vi "Vision Processing.vi"(4 "error in (no error)":errorcluster, 7 "Image Size":T3=enum."320x240") -> ()   [LabVIEW 2015]
uses:
  Vision Support Code/Camera Types.ctl
  <vilib>/Rock Robotics/WPI/Camera/WPI_CameraImageSize.ctl
  <vilib>/Rock Robotics/WPI/Camera/WPI_CameraWhite Balance Values.ctl
  <vilib>/Rock Robotics/WPI/Camera/WPI_CameraExposure Values.ctl
  <vilib>/Rock Robotics/WPI/Camera/WPI_CameraFrameRate.ctl
  Robot Global Data.vi
  <vilib>/vision/NI_Vision_Development_Module.lvlib
panel:
  out "Highest Avg Score":dbl
  in  "Min Score Threshold":i32=75
  out "Detected Targets":T1(array[cluster]) {"Normalized Rect"."Numeric 5" format="%#_2g"; "Normalized Rect"."Numeric 3" format="%#_2g"; "Normalized Rect"."Numeric 2" format="%#_2g"; "Normalized Rect"."Numeric" format="%#_2g"}
  out "Sorted Particle Scores":T2(array[cluster]) {"Moment Factor" format="%#_3g"; "Aspect Ratio" format="%#_3g"; "Area to CH" format="%#_3g"; "X" format="%#_3g"; "Y" format="%#_3g"}
  in  "Display Original":bool=TRUE
  in  "Display Mask":bool=TRUE
  out "fps":dbl
  in  "Emphasize Limit Tests":bool=TRUE
  in  "Camera Type":T4=enum."MS HD3000 square"
  in  "Aspect Fudge Factor":dbl=1.0
  in  "Score Threshold":dbl=75.0
  out "ms to process":u32
  out "Qualified Particles":i32
  in  "LED Color":T5={"Hue"={79.29295672286403, 141.76422489711763}, "Sat"={66.78571428571429, 255.0}, "Val"={48.571428571428584, 255.0}} {"Hue" scale=0.0..255.0 scale format="%#_3g"}
  out "Masked":T6(plugin-control)
  out "Original Image":T6(plugin-control)
  # "This is only the initial camera size.\nOther camera setup is done\non the diagram. Notice it is set\nonce before the loop but can be\nupdated within the loop if needed."
  # "Instructions:\nUse LED Color to threshold and build particles. Adjust calibration if needed.\nDisplays are very useful for debugging, but will slow down execution, so you\nmay want to disable once working.\nAnnotations show the rectangle and the scores from top to bottom.\nChange camera setting on diagram."
  # "Density Profile"
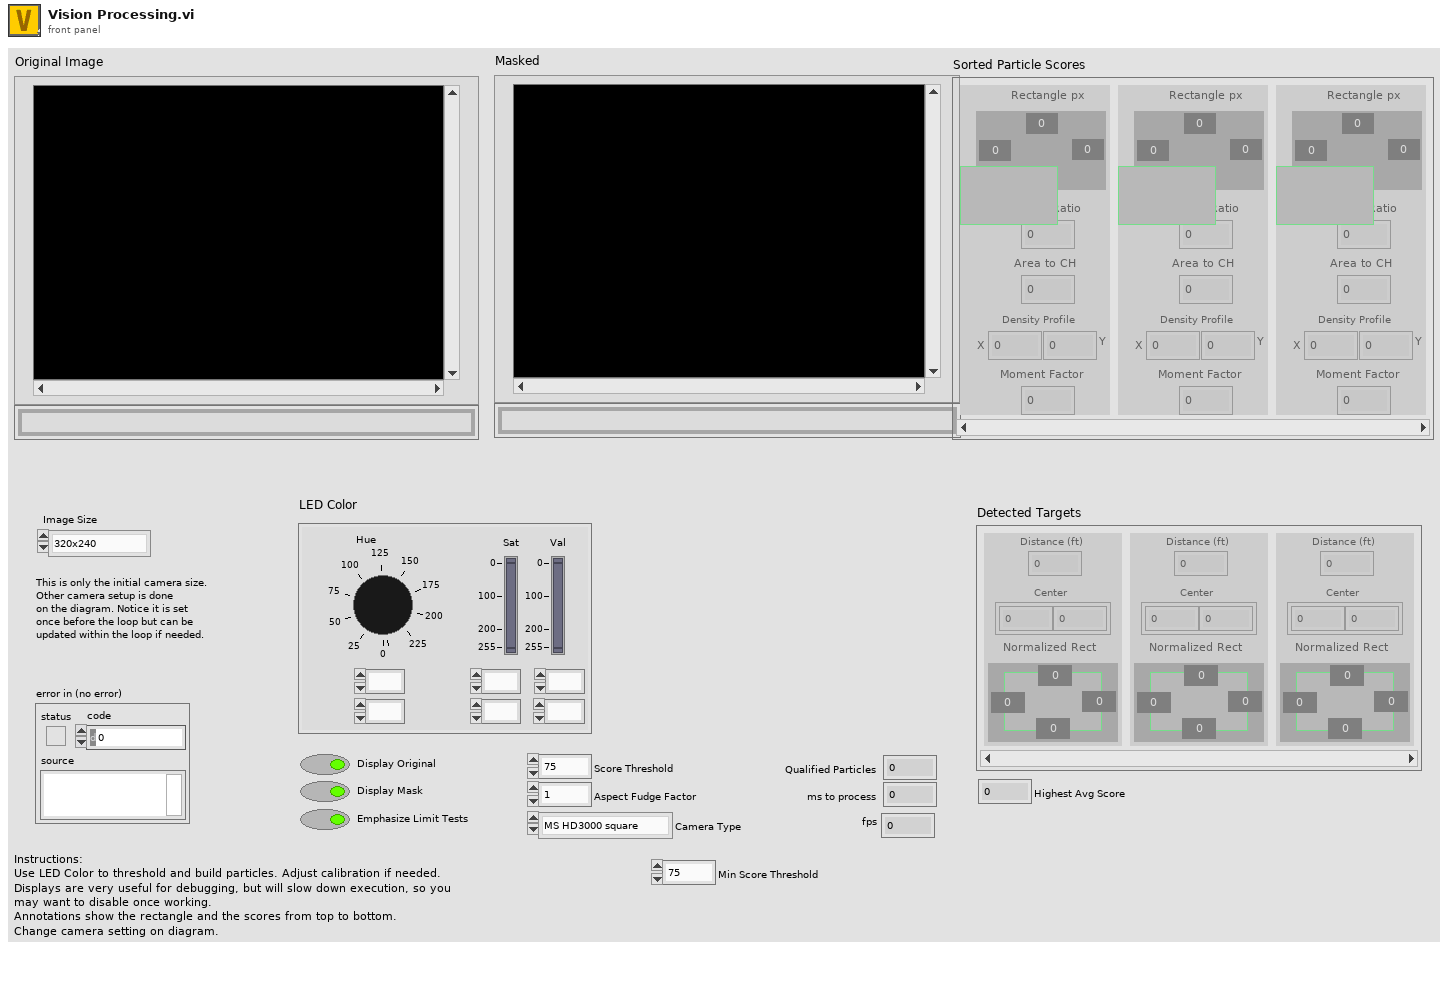
[diagram p1: front panel]
types:
  T1 = cluster{"Distance (ft)":dbl, "Center":cluster{dbl, dbl}, "Normalized Rect":cluster{"Numeric":dbl, "Numeric 2":dbl, "Numeric 3":dbl, "Numeric 5":dbl}}[]
  T2 = cluster{"Rectangle px":cluster{"Numeric":dbl, "Numeric 2":dbl, "Numeric 3":dbl, "Numeric 5":dbl}, "Aspect Ratio":dbl, "Area to CH":dbl, "X":dbl, "Y":dbl, "Moment Factor":dbl}[]
  T3 = typedef "WPI_CameraImageSize.ctl" = enum16{"640x480", "320x240", "160x120", "Custom"}
  T4 = typedef "Camera Types.ctl" = enum16{"206", "1011", "1013", "MS HD3000 square", "MS HD3000 640x480"}
  T5 = cluster{"Hue":cluster{dbl, dbl}, "Sat":cluster{dbl, dbl}, "Val":cluster{dbl, dbl}}
  T6 = typedef "IMAQ Image.ctl" = refnum<image>
  T7 = typedef "WPI_CameraFrameRate.ctl" = u32
  T8 = typedef "WPI_CameraExposure Values.ctl" = enum16{"Auto", "Flicker-free 50 Hz", "Flicker-free 60 Hz", "Hold current", "Custom"}
  T9 = typedef "WPI_CameraWhite Balance Values.ctl" = enum16{"Auto", "Fixed indoor", "Fixed outdoor 1", "Fixed outdoor 2", "Fixed fluorescent 1", "Fixed fluorescent 2", "Hold current", "Custom"}
  T10 = typedef "Particle Parameters" = i32
  T11 = typedef "Image Type" = u32
  T12 = typedef "WPI_CameraDevRef.ctl" = cluster{"Camera Address":string, "CameraStatus":errorcluster}
  T13 = cluster{"Bounding box":cluster{"left":dbl, "top":dbl, "right":dbl, "bottom":dbl}, "Aspect Ratio":dbl, "Area to CH":dbl, "X Mask":dbl, "Y Mask":dbl, "Moment":dbl}[]
  T14 = cluster{"Rectangle":cluster{"Numeric":dbl, "Numeric 2":dbl, "Numeric 3":dbl, "Numeric 5":dbl}, "L":dbl, "Area to CH":dbl, "X":dbl, "Y":dbl, "Moment Factor":dbl}[]
  T15 = cluster{"Found Targets[0]":cluster{"Distance (ft)":dbl, "Center":cluster{dbl, dbl}, "Normalized Rect":cluster{"Numeric":dbl, "Numeric 2":dbl, "Numeric 3":dbl, "Numeric 5":dbl}}, "Found Targets[1]":cluster{"Distance (ft)":dbl, "Center":cluster{dbl, dbl}, "Normalized Rect":cluster{"Numeric":dbl, "Numeric 2":dbl, "Numeric 3":dbl, "Numeric 5":dbl}}, "Found Targets[2]":cluster{"Distance (ft)":dbl, "Center":cluster{dbl, dbl}, "Normalized Rect":cluster{"Numeric":dbl, "Numeric 2":dbl, "Numeric 3":dbl, "Numeric 5":dbl}}, "Found Targets[3]":cluster{"Distance (ft)":dbl, "Center":cluster{dbl, dbl}, "Normalized Rect":cluster{"Numeric":dbl, "Numeric 2":dbl, "Numeric 3":dbl, "Numeric 5":dbl}}, "Found Targets[4]":cluster{"Distance (ft)":dbl, "Center":cluster{dbl, dbl}, "Normalized Rect":cluster{"Numeric":dbl, "Numeric 2":dbl, "Numeric 3":dbl, "Numeric 5":dbl}}, "Found Targets[5]":cluster{"Distance (ft)":dbl, "Center":cluster{dbl, dbl}, "Normalized Rect":cluster{"Numeric":dbl, "Numeric 2":dbl, "Numeric 3":dbl, "Numeric 5":dbl}}, "Found Targets[6]":cluster{"Distance (ft)":dbl, "Center":cluster{dbl, dbl}, "Normalized Rect":cluster{"Numeric":dbl, "Numeric 2":dbl, "Numeric 3":dbl, "Numeric 5":dbl}}, "Found Targets[7]":cluster{"Distance (ft)":dbl, "Center":cluster{dbl, dbl}, "Normalized Rect":cluster{"Numeric":dbl, "Numeric 2":dbl, "Numeric 3":dbl, "Numeric 5":dbl}}, "Found Targets[8]":cluster{"Distance (ft)":dbl, "Center":cluster{dbl, dbl}, "Normalized Rect":cluster{"Numeric":dbl, "Numeric 2":dbl, "Numeric 3":dbl, "Numeric 5":dbl}}}
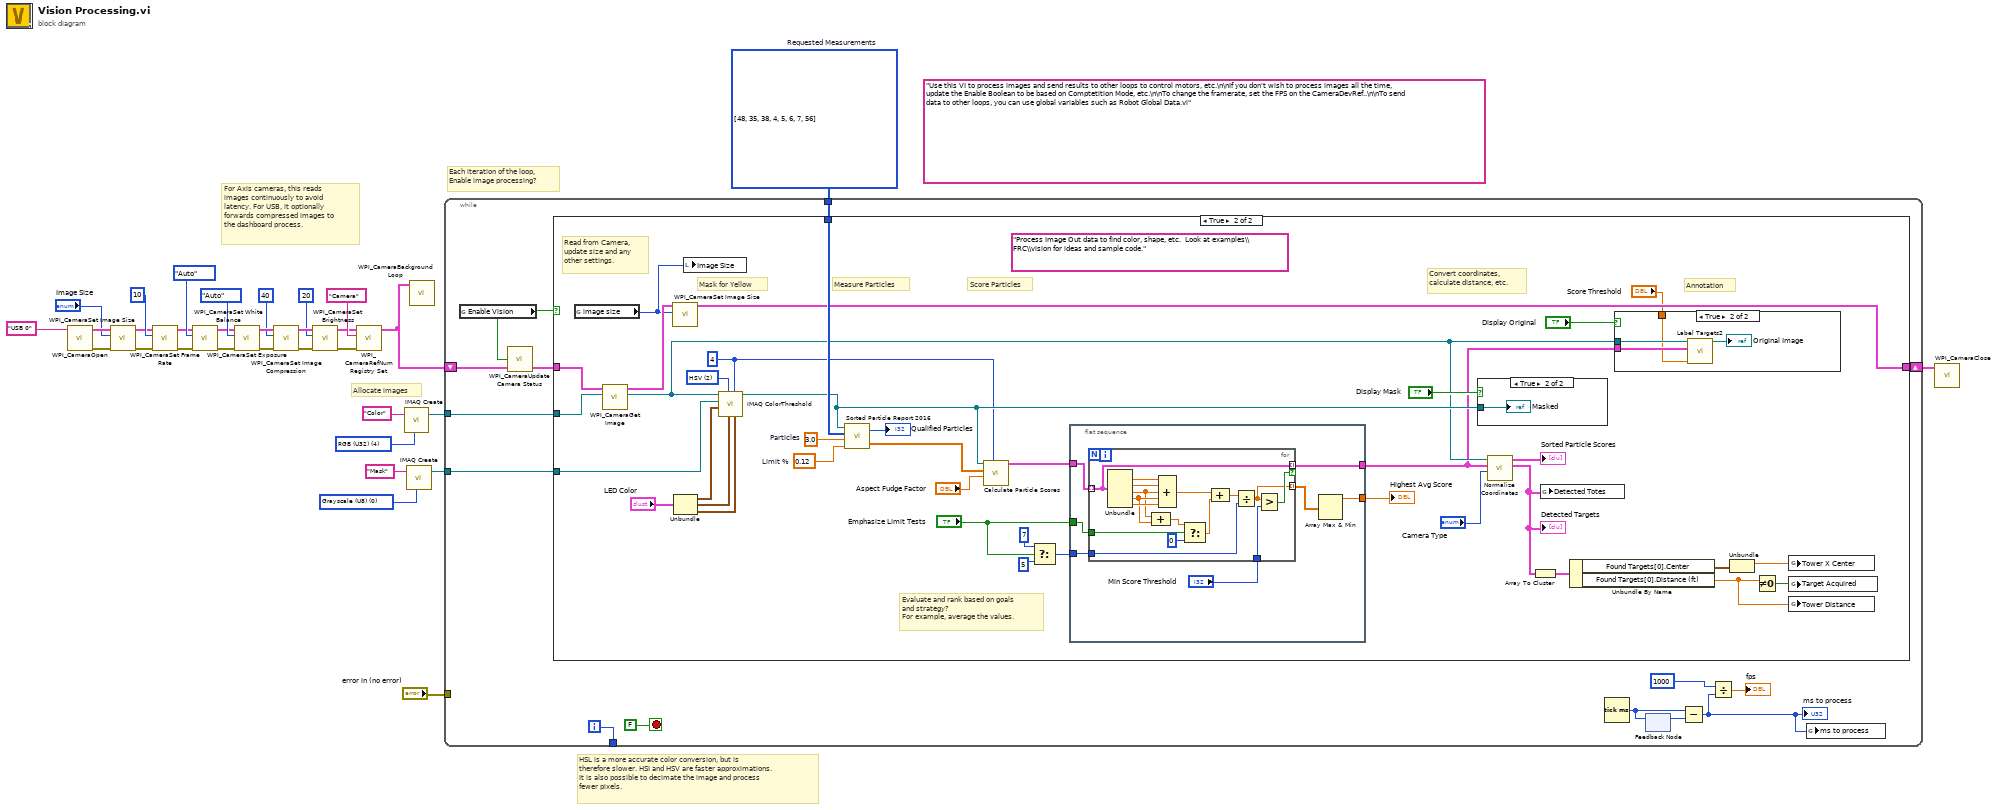
[diagram p0: block diagram]
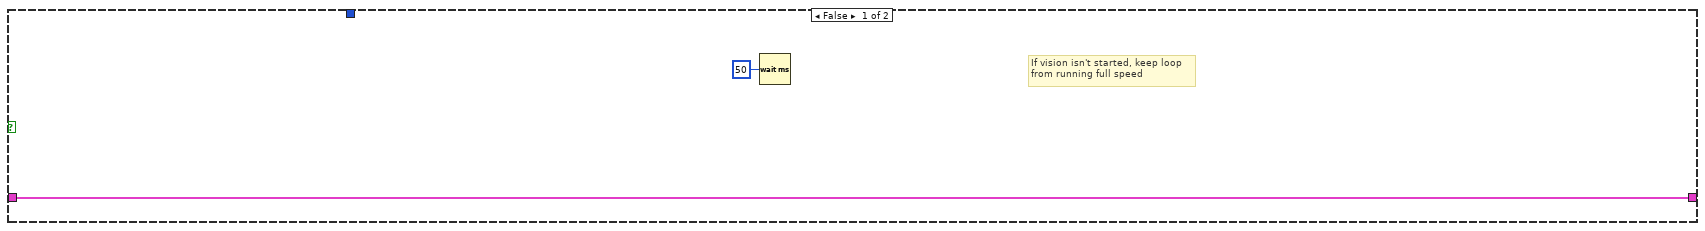
[diagram p2: hidden frame]
diagram:
  (unwired) "Use this VI to process images and send results to other loops to control motors, etc.\n\nIf you don't wish to process images all the time, update the Enable Boolean to be based on Comptetition Mode, etc.\n\nTo change the framerate, set the FPS on the CameraDevRef..\n\nTo send data to other loops, you can use global variables such as Robot Global Data.vi"
  w26 = T10[] [48, 35, 38, 4, 5, 6, 7, 56] items=["Center of Mass X", "Center of Mass Y", "First Pixel X", "First Pixel Y", "Bounding Rect Left", "Bounding Rect Top", "Bounding Rect Right", "Bounding Rect Bottom", "Max Feret Diameter Start X", "Max Feret Diameter Start Y", "Max Feret Diameter End X", "Max Feret Diameter End Y", "Max Horiz. Segment Length Left", "Max Horiz. Segment Length Right", "Max Horiz. Segment Length Row", "-", "Bounding Rect Width", "Bounding Rect Height", "Bounding Rect Diagonal", "Perimeter", "Convex Hull Perimeter", "Holes' Perimeter", "Max Feret Diameter", "Equivalent Ellipse Major Axis", "Equivalent Ellipse Minor Axis", "Equivalent Ellipse Minor Axis (Feret)", "Equivalent Rect Long Side", "Equivalent Rect Short Side", "Equivalent Rect Diagonal", "Equivalent Rect Short Side (Feret)", "Average Horiz. Segment Length", "Average Vert. Segment Length", "Hydraulic Radius", "Waddel Disk Diameter", "-", "Area", "Holes' Area", "Particle & Holes' Area", "Convex Hull Area", "Image Area", "-", "Number of Holes", "Number of Horiz. Segments", "Number of Vert. Segments", "-", "Orientation", "Max Feret Diameter Orientation", "-", "% Area/Image Area", "% Area/(Particle & Holes' Area)", "Ratio of Equivalent Ellipse Axes", "Ratio of Equivalent Rect Sides", "-", "Elongation Factor", "Compactness Factor", "Heywood Circularity Factor", "Type Factor", "-", "Sum X", "Sum Y", "Sum XX", "Sum XY", "Sum YY", "Sum XXX", "Sum XXY", "Sum XYY", "Sum YYY", "-", "Moment of Inertia XX", "Moment of Inertia XY", "Moment of Inertia YY", "Moment of Inertia XXX", "Moment of Inertia XXY", "Moment of Inertia XYY", "Moment of Inertia YYY", "Norm. Moment of Inertia XX", "Norm. Moment of Inertia XY", "Norm. Moment of Inertia YY", "Norm. Moment of Inertia XXX", "Norm. Moment of Inertia XXY", "Norm. Moment of Inertia XYY", "Norm. Moment of Inertia YYY", "Hu Moment 1", "Hu Moment 2", "Hu Moment 3", "Hu Moment 4", "Hu Moment 5", "Hu Moment 6", "Hu Moment 7"]  # Requested Measurements
  w29 = T11 0 items=["Grayscale (U8)", "Grayscale (I16)", "Grayscale (SGL)", "Complex (CSG)", "RGB (U32)", "HSL (U32)", "RGB (U64)", "Grayscale (U16)"] ("Image Type")
  w31 = T11 4 items=["Grayscale (U8)", "Grayscale (I16)", "Grayscale (SGL)", "Complex (CSG)", "RGB (U32)", "HSL (U32)", "RGB (U64)", "Grayscale (U16)"] ("Image Type")
  # "Each iteration of the loop,\nEnable image processing?"
  # "HSL is a more accurate color conversion, but is\ntherefore slower. HSI and HSV are faster approximations.\nIt is also possible to decimate the image and process\nfewer pixels."
  # "For Axis cameras, this reads\nimages continuously to avoid\nlatency. For USB, it optionally\nforwards compressed images to\nthe dashboard process."
  # "Allocate images"
  n1 = call <vilib>:"WPI_CameraOpen.vi"("Camera Address"="USB 0" ("format string")) -> ("error out"=w16:errorcluster, "CameraDevRef"=w15:T12)  [unwired: 1 in, 8 out]
  n2 = call <vilib>:"WPI_CameraSet Image Size.vi"("error in (no error)"=w16, "Image Size"="Image Size", "CameraDevRef"=w15) -> ("error out"=w17:errorcluster, "CameraDevRef Out"=w14:T12)  [unwired: 1 in, 6 out]
  n3 = call <vilib>:"WPI_CameraSet Frame Rate.vi"("error in (no error)"=w17, "Frame Rate (fps)"=T7 10, "CameraDevRef"=w14) -> ("error out"=w18:errorcluster, "CameraDevRef Out"=w12:T12)  [unwired: 7 out]
  n4 = call <vilib>:"WPI_CameraSet White Balance.vi"("error in (no error)"=w18, "White Balance"=WPI_CameraWhite_Balance_Values."Auto", "CameraDevRef"=w12) -> ("error out"=w19:errorcluster, "CameraDevRef Out"=w13:T12)  [unwired: 1 in, 6 out]
  n5 = call <vilib>:"WPI_CameraSet Exposure.vi"("error in (no error)"=w19, "Exposure"=WPI_CameraExposure_Values."Auto", "CameraDevRef"=w13) -> ("error out"=w20:errorcluster, "CameraDevRef Out"=w10:T12)  [unwired: 1 in, 6 out]
  n6 = call <vilib>:"WPI_CameraSet Image Compression.vi"("error in (no error)"=w20, "Compression"=40, "CameraDevRef"=w10) -> ("error out"=w21:errorcluster, "CameraDevRef Out"=w11:T12)  [unwired: 7 out]
  n7 = call <vilib>:"WPI_CameraSet Brightness.vi"("error in (no error)"=w21, "Brightness"=20, "CameraDevRef"=w11) -> ("error out"=w22:errorcluster, "CameraDevRef Out"=w2:T12)  [unwired: 7 out]
  n8 = call <vilib>:"WPI_CameraRefNum Registry Set.vi"("error in (no error)"=w22, "refnum name"="Camera", "CameraDevRef"=w2) -> ("CameraDevRef"=w6:T12)  [unwired: 1 in, 7 out]
  n9 = call "IMAQ Create"("Image Name"="Color", "Image Type"=w31) -> ("New Image"=w30:T6)  [unwired: 2 in, 2 out]
  n10 = call "IMAQ Create"("Image Name"="Mask", "Image Type"=w29) -> ("New Image"=w27:T6)  [unwired: 2 in, 2 out]
  n11 = call <vilib>:"WPI_CameraBackground Loop.vi"("CameraDevRef"=w6) -> ()  [unwired: 11 in]
  n12 = while {
    tunnel: w30 -> [w41]
    tunnel: w27 -> [w45]
    tunnel: w26 -> [w44]
    tunnel: "error in (no error)" -> [_]
    tunnel: [w40] -> _
    shift-right: [w36] -> w3
    shift-left: w6 -> [w38]
    i -> [w40]
    stop <- FALSE stop-if-true
    n13 = global read "Robot Global Data.vi" "Enable Vision"() -> (w39:bool)
    n14 = call <vilib>:"WPI_CameraUpdate Camera Status.vi"("CameraDevRef In"=w38, "Enable Vision"=w39) -> ("CameraDevRef Out"=w37:T12)  [unwired: 3 in]
    n15 = case shown="True" w39 {
      tunnel: w45 -> [_ w86]
      tunnel: w44 -> [_ w81]
      tunnel: w37 -> [w47 w77]
      tunnel: w41 -> [_ w76]
      tunnel: [w47 w74] -> w36
      frame False {
        # "If vision isn't started, keep loop\nfrom running full speed"
        n16 = Wait (ms)(milliseconds to wait=u32 50) -> ()  [unwired: 1 out]
      }
      frame True {
        w58 = 4 ("Replace Value")
        w71 = u16 2 items=["RGB", "HSL", "HSV", "HSI"] ("Color Mode")
        (unwired) "Process Image Out data to find color, shape, etc.  Look at examples\\FRC\\vision for ideas and sample code."
        w78 = 0.12  # Limit %
        w80 = 3.0  # Particles
        # "Evaluate and rank based on goals\nand strategy?\nFor example, average the values."
        # "Read from Camera,\nupdate size and any\nother settings."
        # "Measure Particles"
        # "Convert coordinates,\ncalculate distance, etc."
        # "Annotation"
        # "Score Particles"
        # "Mask for Yellow"
        n17 = global read "Robot Global Data.vi" "image size"() -> (w57:T3)
        n18 = call <vilib>:"WPI_CameraGet Image.vi"("Image"=w76, "CameraDevRef"=w77) -> ("Image Out"=w61:T6, "CameraDevRef Out"=w75:T12)  [unwired: 7 in, 1 out]
        n19 = call <vilib>:"WPI_CameraSet Image Size.vi"("Image Size"=w57, "CameraDevRef"=w75) -> ("CameraDevRef Out"=w74:T12)  [unwired: 2 in, 7 out]
        n20 = Unbundle("LED Color") -> ("Hue"=w85:cluster{dbl, dbl}, "Sat"=w84:cluster{dbl, dbl}, "Val"=w83:cluster{dbl, dbl})
        n21 = local write "Image Size"(w57) -> ()
        n22 = call "IMAQ ColorThreshold"("Blue or Luma or Val or Inten Range"=w83, "Replace Value"=w58, "Green or Sat Range"=w84, "Color Mode"=w71, "Red or Hue Range"=w85, "Image Dst"=w86, "Image Src"=w61) -> ("Image Dst Out"=w70:T6)  [unwired: 3 in, 1 out]
        n23 = call "Sorted Particle Report 2016.vi"("Min Area Size %"=w78, "Particle Count Limit"=w80, "Pixel Measurements"=w81, "Image in"=w70) -> ("Sorted Data"=w69:dbl[][], "Particles"=→"Qualified Particles":i32)
        n24 = call "Calculate Particle Scores.vi"("Pixel Value"=w58, "Aspect Fudge Factor"="Aspect Fudge Factor", "Sorted Data"=w69, "Image in"=w70) -> ("Scores"=w67:T13)  [unwired: 7 in]
        n25 = Select(t=7, s="Emphasize Limit Tests", f=5) -> (s? t:f=w64:i32)
        n26 = flat-sequence {
          tunnel: w67 -> [w97]
          tunnel: w64 -> [w95]
          tunnel: [w98] -> w63
          tunnel: [w92] -> w60
          tunnel: "Emphasize Limit Tests" -> [w96]
          frame #0 {
            n27 = for {
              tunnel: w97 -> [w112] mode=indexing
              tunnel: [w112] -> w92 mode=indexing if=w111
              tunnel: [w110] -> w93 mode=indexing
              tunnel: w95 -> [w109]
              tunnel: "Min Score Threshold" -> [w108]
              tunnel: w96 -> [w101]
              n28 = Unbundle(w112) -> ("Aspect Ratio"=w114:dbl, "Area to CH"=w113:dbl, "X Mask"=w103:dbl, "Y Mask"=w104:dbl, "Moment"=w105:dbl)  [unwired: 1 out]
              n29 = Compound Arithmetic op=ADD(w103, w104) -> (w102:dbl)
              n30 = Compound Arithmetic op=ADD(w114, w113, w103, w104, w105) -> (w107:dbl)
              n31 = Select(t=w102, s=w101, f=0) -> (s? t:f=w100:dbl)
              n32 = Compound Arithmetic op=ADD(w107, w100) -> (w106:dbl)
              n33 = Divide(x=w106, y=w109) -> (x/y=w110:dbl)
              n34 = Greater?(x=w110, y=w108) -> (0:w111:bool)
            }
            n35 = Array Max & Min(array=w93) -> (max value=w98:dbl)  [unwired: 3 out]
          }
        }
        n36 = case shown="True" "Display Mask" {
          tunnel: w70 -> [_ w91]
          frame False {
          }
          frame True {
            "Masked" <- w91
          }
        }
        n37 = call "Normalize Coordinates.vi"("Camera Type"="Camera Type", "Targets"=w60, "Image in"=w61) -> ("Found Targets"=w53:T1, "Sorted Scores"=→"Sorted Particle Scores":T14)  [unwired: 7 in]
        "Detected Targets" <- w53
        n38 = Array To Cluster(array=w53) -> (cluster=w55:T15)
        n39 = global write "Robot Global Data.vi" "Detected Totes"(w53) -> ()
        n40 = Unbundle By Name(w55) -> ("Found Targets[0].Center"=w51:cluster{dbl, dbl}, "Found Targets[0].Distance (ft)"=w49:dbl)
        n41 = case shown="True" "Display Original" {
          tunnel: w61 -> [_ w90]
          tunnel: w60 -> [_ w88]
          tunnel: "Score Threshold" -> [_ w87]
          frame False {
          }
          frame True {
            n42 = call "Label Targets2.vi"("Score Threshold"=w87, "Targets"=w88, "Image in"=w90) -> ("Image out"=→"Original Image":T6)  [unwired: 8 in]
          }
        }
        n43 = Unbundle(w51) -> (w50:dbl)  [unwired: 1 out]
        n44 = Not Equal To 0?(x=w49) -> (x != 0?=w52:bool)
        n45 = global write "Robot Global Data.vi" "Tower X Center"(w50) -> ()
        n46 = global write "Robot Global Data.vi" "Target Acquired"(w52) -> ()
        n47 = global write "Robot Global Data.vi" "Tower Distance"(w49) -> ()
        "Highest Avg Score" <- w63
      }
    }
    n48 = Tick Count (ms)() -> (millisecond timer value=w42:u32)
    n49 = feedback-in #1(w42) -> ()
    n50 = feedback #1() -> (w43:u32)  [unwired: 1 in]
    n51 = Subtract(x=w42, y=w43) -> (x-y=w35:u32)
    "ms to process" <- w35
    n52 = Divide(x=1000 ("Brightness"), y=w35) -> (x/y=→"fps":dbl)
    n53 = global write "Robot Global Data.vi" "ms to process"(w35) -> ()
  }
  n54 = call <vilib>:"WPI_CameraClose.vi"("CameraDevRef"=w3) -> ()  [unwired: 1 in, 10 out]
